vi "SUB-Text_Blink.vi"(7 "Timeout":dbl=3.0, 9 "text color":u32, 10 "Stop":bool, 11 "Message":string) -> ()   [LabVIEW 2015]
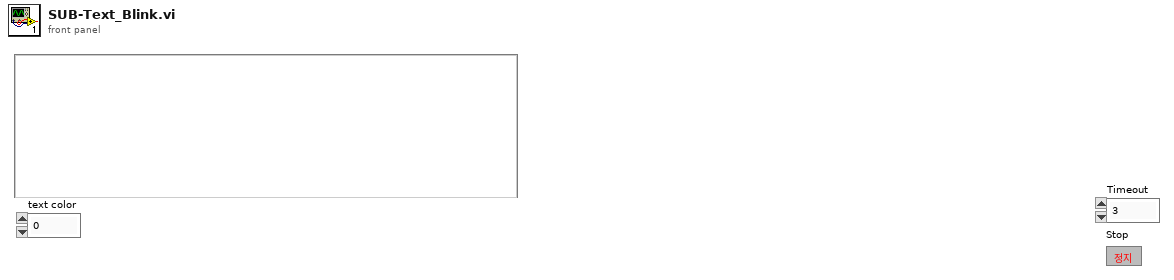
[diagram p1: front panel]
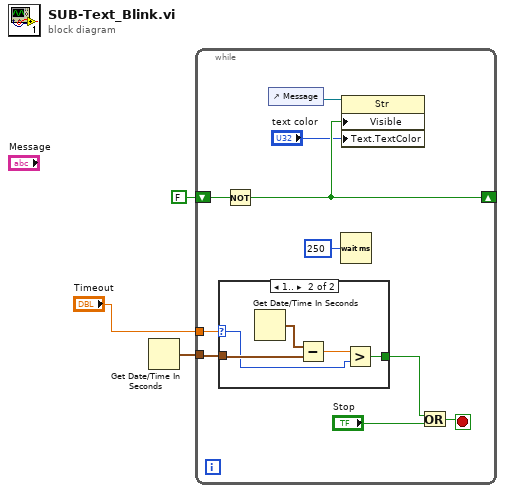
[diagram p0: block diagram]
diagram:
  n1 = Get Date/Time In Seconds() -> (seconds since 1Jan1904=w2:timestamp)
  n2 = while {
    shift-right: [w11] -> _
    shift-left: FALSE -> [w12]
    tunnel: w2 -> [w9]
    tunnel: "Timeout" -> [w8]
    stop <- w7 stop-if-true
    n3 = case shown="1.." w8 {
      selector: w8 -> [_ w15]
      tunnel: w9 -> [_ w17]
      tunnel: [_ w14] -> w5
      frame 0, Default {
      }
      frame 1.. {
        n4 = Get Date/Time In Seconds() -> (seconds since 1Jan1904=w18:timestamp)
        n5 = Subtract(x=w18, y=w17) -> (x-y=w16:dbl)
        n6 = Greater?(x=w16, y=w15) -> (0:w14:bool)
      }
    }
    n7 = Not(x=w12) -> (.not. x?=w11:bool)
    n8 = control-ref of="Message"() -> (w13:refnum<vi>)
    n9 = Wait (ms)(milliseconds to wait=u32 250 ("대기 시간(ms)")) -> ()  [unwired: 1 out]
    n10 = property class="Str"(reference=w13, "Visible"=w11, "Text.TextColor"="text color") -> ()  [unwired: 1 in, 2 out]
    n11 = Or(x=w5, y="Stop") -> (x .or. y?=w7:bool)
  }
